vi "Custom.vi"(8 "error in (no error)":errorcluster) -> (0 "error out":errorcluster)   [LabVIEW 2020, in "FirmataClient.lvlib"]
doc: "Allows sending custom messages to the board. Enter the message as hex separated with \"-\" (i.e. to request firrmware, enter \"F0-79-F7\" and expect \"F0-79-2-5-53-0-74-0-61-0-6E-0-64-0-61-0-72-0-64-0-46-0-69-0-72-0-6D-0-61-0-74-0-61-0-2E-0-69-0-6E-0-6F-0-F7\" as \"StandardFirmata.ino and v2.5\")."
uses:
  FirmataClient.lvlib
  Controls/SupportedTransports.ctl
panel:
  in  "Connection Details":enum32{"Serial Communication", "Page 2"}(tab)
  in  "Baud Rate":u32(ring)=57600 items=["75"=75, "110"=110, "134"=134, "150"=150, "300"=300, "600"=600, "1200"=1200, "1800"=1800, "2400"=2400, "4800"=4800, "7200"=7200, "9600"=9600, "14400"=14400, "19200"=19200, "28800"=28800, "38400"=38400, "56000"=56000, "57600"=57600, "115200"=115200, "128000"=128000, "230400"=230400]
  in  "Comport":refnum<visa-resource-name>="COM20"
  in  "Select Transport Mode":T1
  in  "Message In":string="F0-79-F7"
  out "Response":string
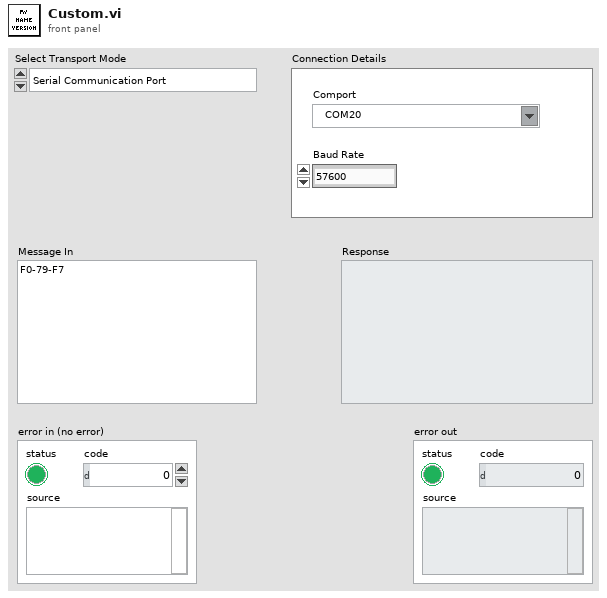
[diagram p1: front panel]
types:
  T1 = typedef "FirmataClient.lvlib/SupportedTransports.ctl" = enum16{"Serial Communication Port"}
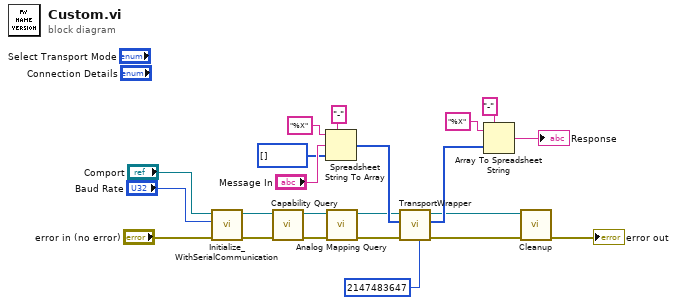
[diagram p0: block diagram]
diagram:
  n1 = call "Initialize_WithSerialCommunication.vi"("error in"="error in (no error)", "Baud Rate"="Baud Rate", "Comport"="Comport") -> ("error out"=w12:errorcluster, "Refnum Out"=w13:refnum<vi>)  [unwired: 4 in, 3 out]
  n2 = call "Capability Query.vi"("error in (no error)"=w12, "Refnum In"=w13) -> ("error out"=w10:errorcluster, "Refnum Out"=w11:refnum<vi>)  [unwired: 7 in, 1 out]
  n3 = Spreadsheet String To Array(delimiter (Tab)="-", format string="%X", spreadsheet string="Message In", array type (2D Dbl)=u8[] []) -> (array=w15:u8[])
  n4 = call "Analog Mapping Query.vi"("error in (no error)"=w10, "Refnum In"=w11) -> ("error out"=w8:errorcluster, "Refnum Out"=w7:refnum<vi>)  [unwired: 7 in, 1 out]
  n5 = call "TransportWrapper.vi"("ReplyLength"=2147483647, "error in"=w8, "Message In"=w15, "Refnum In"=w7) -> ("error out"=w6:errorcluster, "Message Out"=w14:u8[], "Refnum Out"=w4:refnum<vi>)  [unwired: 5 in]
  n6 = Array To Spreadsheet String(delimiter (Tab)="-", array=w14, 3:"%X" ("format string")) -> (spreadsheet string=→"Response":string)
  n7 = call "Cleanup.vi"("error in"=w6, "Refnum In"=w4) -> ("error out"=→"error out":errorcluster)  [unwired: 9 in]
